vi "openTDMS.vi"(8 "error in (no error)":errorcluster {"code" format="Error %.0f"}, 11 "tdmsFilepath":path) -> (0 "error out":errorcluster {"code" format="Error %.0f"}, 3 "tdmsRef":refnum<k34>)   [LabVIEW 2017]
doc: "This VI creates or opens a TDMS file and appends a timestamp to the filename."
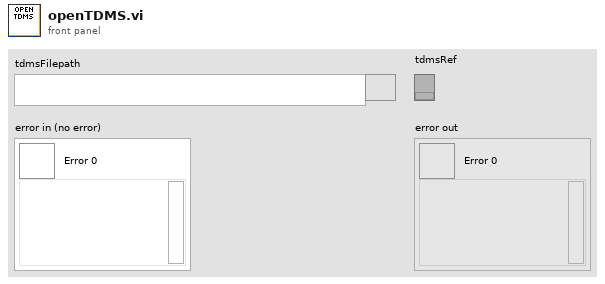
[diagram p1: front panel]
types:
  T1 = enum16{"open", "open or create", "create or replace", "create", "open (read-only)"}
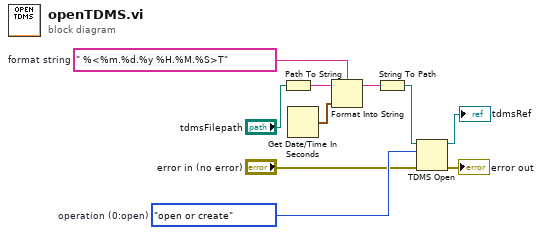
[diagram p0: block diagram]
diagram:
  w6 = " %<%m.%d.%y %H.%M.%S>T"  # format string
  w8 = T1."open or create"  # operation (0:open)
  n1 = Path To String(path="tdmsFilepath") -> (string=w5:string)
  n2 = Get Date/Time In Seconds() -> (seconds since 1Jan1904=w7:timestamp)
  n3 = Format Into String(format string=w6, initial string=w5, w7) -> (resulting string=w4:string)  [unwired: 1 in, 1 out]
  n4 = String To Path(string=w4) -> (path=w9:path)
  n5 = TDMS Open(8:"error in (no error)", 10:w8, 11:w9) -> (0:→"error out":errorcluster, 3:→"tdmsRef":refnum<k34>)  [unwired: 4 in]
